vi "Rising Edge Trigger.vi"(1 "Raw Signal":bool) -> (0 "Trigger":bool)   [LabVIEW 2018]
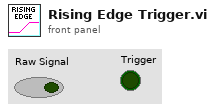
[diagram p1: front panel]
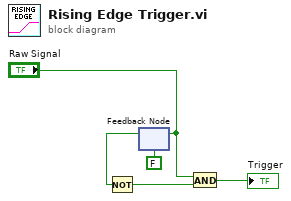
[diagram p0: block diagram]
diagram:
  n1 = feedback-in #1("Raw Signal") -> ()
  n2 = feedback #1(FALSE ("Raw Signal")) -> (w5:bool)
  n3 = Not(x=w5) -> (.not. x?=w3:bool)
  n4 = And(x="Raw Signal", y=w3) -> (x .and. y?=→"Trigger":bool)
